vi "XML readSamplesFromXML.vi"(11 "Samples (XML)":string[](array[string])) -> (3 "Sample":T1[](array[typedef]))   [LabVIEW 2011]
uses:
  Controls/PIM.API.Response.Samples.ctl
  iQA Sweep Behavior.ctl
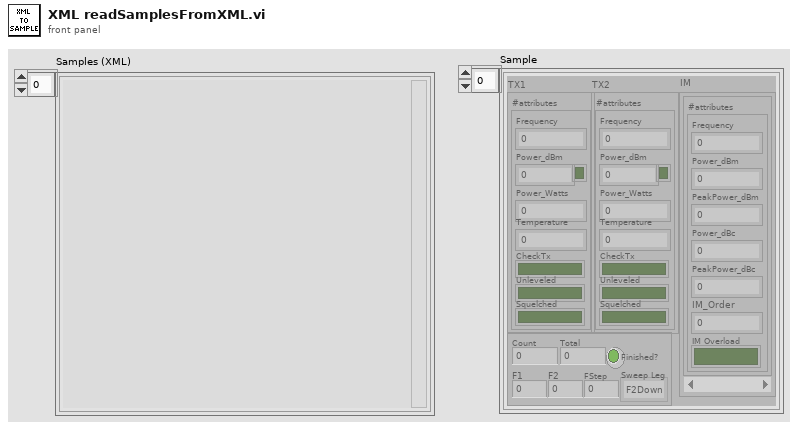
[diagram p1: front panel]
types:
  T1 = typedef "PIM.API.Response.Samples.ctl" = cluster{"TX1":cluster{"#attributes":cluster{"Frequency":dbl, "Power_dBm":dbl, "Power_Watts":dbl, "CheckTx":bool, "Unleveled":bool, "Squelched":bool, "Temperature":dbl, "ToneOn":bool}}, "TX2":cluster{"#attributes":cluster{"Frequency":dbl, "Power_dBm":dbl, "Power_Watts":dbl, "CheckTx":bool, "Unleveled":bool, "Squelched":bool, "Temperature":dbl, "ToneOn":bool}}, "IM":cluster{"#attributes":cluster{"Frequency":dbl, "Power_dBm":dbl, "PeakPower_dBm":dbl, "Power_dBc":dbl, "PeakPower_dBc":dbl, "IM_Order":u8, "IM Overload":bool}}[], "#attributes":cluster{"Count":u32, "Total":u32, "Finished?":bool, "Sweep Leg":T2, "F1":dbl, "F2":dbl, "FStep":dbl}}
  T2 = typedef "iQA Sweep Behavior.ctl" = enum16{"F2Down", "F1Up", "RxMultiIM"}
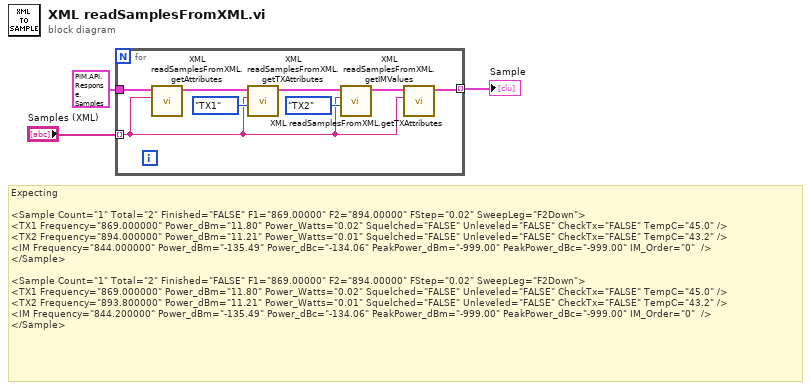
[diagram p0: block diagram]
diagram:
  # "Expecting\n\n<Sample Count=\"1\" Total=\"2\" Finished=\"FALSE\" F1=\"869.00000\" F2=\"894.00000\" FStep=\"0.02\" SweepLeg=\"F2Down\">\n<TX1 Frequency=\"869.000000\" Power_dBm=\"11.80\" Power_Watts=\"0.02\" Squelched=\"FALSE\" Unleveled=\"FALSE\" CheckTx=\"FALSE\" TempC=\"45.0\" />\n<TX2 Frequency=\"894.000000\" Power_dBm=\"11.21\" Power_Watts=\"0.01\" Squelched=\"FALSE\" Unleveled=\"FALSE\" CheckTx=\"FALSE\" TempC=\"43.2\" />\n<IM Frequency=\"844.000000\" Power_dBm=\"-135.49\" Power_dBc=\"-134.06\" PeakPower_dBm=\"-999.00\" PeakPower_dBc=\"-999.00\" IM_Order=\"0\"  />\n</Sample>\n\n<Sample Count=\"1\" Total=\"2\" Finished=\"FALSE\" F1=\"869.00000\" F2=\"894.00000\" FStep=\"0.02\" SweepLeg=\"F2Down\">\n<TX1 Frequency=\"869.000000\" Power_dBm=\"11.80\" Power_Watts=\"0.02\" Squelched=\"FALSE\" Unleveled=\"FALSE\" CheckTx=\"FALSE\" TempC=\"45.0\" />\n<TX2 Frequency=\"893.800000\" Power_dBm=\"11.21\" Power_Watts=\"0.01\" Squelched=\"FALSE\" Unleveled=\"FALSE\" CheckTx=\"FALSE\" TempC=\"43.2\" />\n<IM Frequency=\"844.200000\" Power_dBm=\"-135.49\" Power_dBc=\"-134.06\" PeakPower_dBm=\"-999.00\" PeakPower_dBc=\"-999.00\" IM_Order=\"0\"  />\n</Sample>"
  n1 = for {
    tunnel: "Samples (XML)" -> [w6] mode=indexing
    tunnel: T1 {"TX1"={"#attributes"={"Frequency"=0.0, "Power_dBm"=0.0, "Power_Watts"=0.0, "CheckTx"=FALSE, "Unleveled"=FALSE, "Squelched"=FALSE, "Temperature"=0.0, "ToneOn"=FALSE}}, "TX2"={"#attributes"={"Frequency"=0.0, "Power_dBm"=0.0, "Power_Watts"=0.0, "CheckTx"=FALSE, "Unleveled"=FALSE, "Squelched"=FALSE, "Temperature"=0.0, "ToneOn"=FALSE}}, "IM"=[], "#attributes"={"Count"=0, "Total"=0, "Finished?"=FALSE, "Sweep Leg"=enum."F2Down", "F1"=0.0, "F2"=0.0, "FStep"=0.0}} ("Sample") -> [w11]
    tunnel: [w4] -> w1 mode=indexing
    n2 = call "XML readSamplesFromXML.getAttributes.vi"("Sample XML"=w6, "Sample in"=w11) -> ("Sample out"=w10:T1)  [unwired: 9 in]
    n3 = call "XML readSamplesFromXML.getTXAttributes.vi"("TXSelect (TX1"=enum16{"TX1", "TX2"}."TX1", "Sample XML"=w6, "Sample in"=w10) -> ("Sample out"=w7:T1)  [unwired: 8 in]
    n4 = call "XML readSamplesFromXML.getTXAttributes.vi"("TXSelect (TX1"=enum16{"TX1", "TX2"}."TX2", "Sample XML"=w6, "Sample in"=w7) -> ("Sample out"=w5:T1)  [unwired: 8 in]
    n5 = call "XML readSamplesFromXML.getIMValues.vi"("Sample XML"=w6, "Sample in"=w5) -> ("Sample out"=w4:T1)  [unwired: 9 in]
  }
  "Sample" <- w1
